vi "Set DS Reply Variable.vi"(10 "DS Reply Variable":string, 11 "Reply Msg DataSocket in":refnum<class "Reply Msg DataSocket.lvclass">) -> (3 "Reply Msg DataSocket out":refnum<class "Reply Msg DataSocket.lvclass">)   [LabVIEW 2023, in "Reply Msg DataSocket.lvclass"]
uses:
  Reply Msg DataSocket.lvclass
  Reply Msg DataSocket.lvclass/Reply Msg DataSocket.ctl
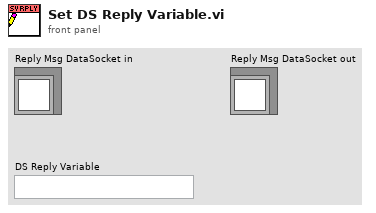
[diagram p1: front panel]
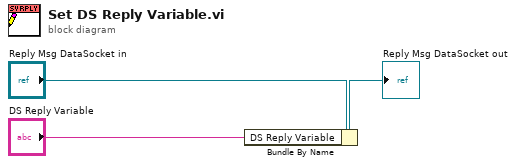
[diagram p0: block diagram]
diagram:
  n1 = Bundle By Name(cluster="Reply Msg DataSocket in", "DS Reply Variable"="DS Reply Variable") -> (→"Reply Msg DataSocket out":refnum<class "Reply Msg DataSocket.lvclass">)
